vi "TCam_ArrayTempExtract.vi"(0 "img in":T1, 7 "Mouse pos":cluster{"X":i32, "Y":i32}, 11 "error in (no error)":errorcluster) -> (3 "Intensity Graph 4":dbl[][](graph), 4 "temp":dbl, 6 "temp str":string, 8 "Mouse pos dup":cluster{"X":i32, "Y":i32}, 15 "error out":errorcluster)   [LabVIEW 2022 SP3]
uses:
  <vilib>/vision/Image Controls.llb/IMAQ Image.ctl
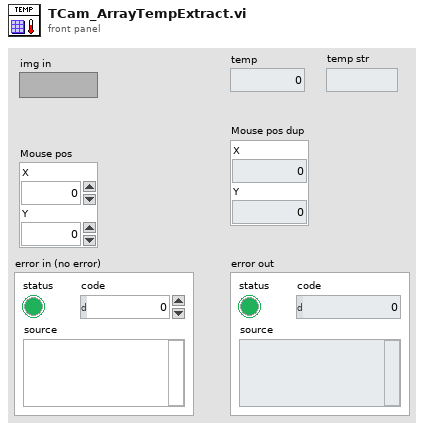
[diagram p1: front panel]
types:
  T1 = typedef "IMAQ Image.ctl" = refnum<image>
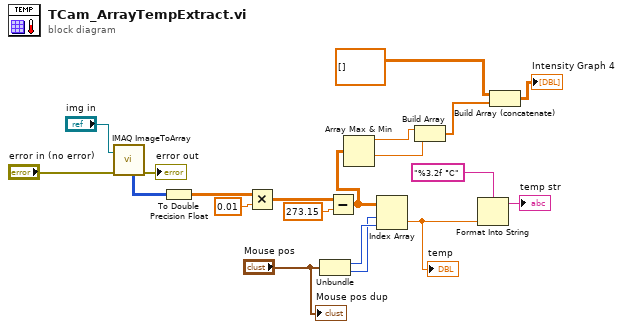
[diagram p0: block diagram]
diagram:
  n1 = call "IMAQ ImageToArray"("error in (no error)"="error in (no error)", "Image"="img in") -> ("Image Pixels (U16)"=w11:u16[][], "error out"=→"error out":errorcluster)  [unwired: 2 in, 3 out]
  n2 = To Double Precision Float(number=w11) -> (double precision float=w14:dbl[][])
  n3 = Multiply(x=w14, y=0.01) -> (x*y=w15:dbl[][])
  n4 = Unbundle("Mouse pos") -> ("X"=w19:i32, "Y"=w18:i32)
  n5 = Subtract(x=w15, y=273.15) -> (x-y=w6:dbl[][])
  n6 = Array Max & Min(array=w6) -> (max value=w2:dbl, min value=w1:dbl)  [unwired: 2 out]
  n7 = Index Array(array=w6, index (row)=w18, index (col)=w19) -> (element=w7:dbl)
  "temp" <- w7
  n8 = Build Array(w2, w1) -> (w3:dbl[])
  n9 = Format Into String(format string="%3.2f °C", w7) -> (resulting string=→"temp str":string)  [unwired: 2 in, 1 out]
  n10 = Build Array (concatenate)(dbl[][] [] ("Intensity Graph 3"), w3) -> (→"Intensity Graph 4":dbl[][])
  "Mouse pos dup" <- "Mouse pos"
